vi "LVClass_WavefrontCorrector Assert Equal User Preferences.vi"(0 "WavefrontCorrector in":refnum<class "WavefrontCorrector.lvclass">, 5 "Wavefront Corrector State":T1[](array[typedef]), 7 "Sleep after command apply (ms)":i32, 11 "error in (no error)":errorcluster) -> (4 "WavefrontCorrector out":refnum<class "WavefrontCorrector.lvclass">, 15 "error out":errorcluster)   [LabVIEW 2020, in "WavefrontCorrector.lvclass"]
doc: "Assert requested preferences are equal to current preferences.\n\n--------------------------------------------------------------------------------\n\n<B>correctorIn </B> : WavefrontCorrector object.\n<B>correctorOut </B> : WavefrontCorrector object.\n<B>sleep_after_movement </B> : WavefrontCorrector preferences : Time to stabilization (ms).\n<B>min </B> : WavefrontCorrector preferences : lowest command value.\n<B>max </B> : WavefrontCorrector preferences : highest command value.\n<B>validity </B> : WavefrontCorrector preferences : status.\n<B>fixed_values </B> : WavefrontCorrector preferences : fixed positions.\n<B>ErrorIn </B> : Error\n<B>ErrorOut </B> : Error\n\n--------------------------------------------------------------------------------"
uses:
  WavefrontCorrector.lvclass
  Wavefront Corrector states - ONE.ctl
  WavefrontCorrector.lvclass/WavefrontCorrector.ctl
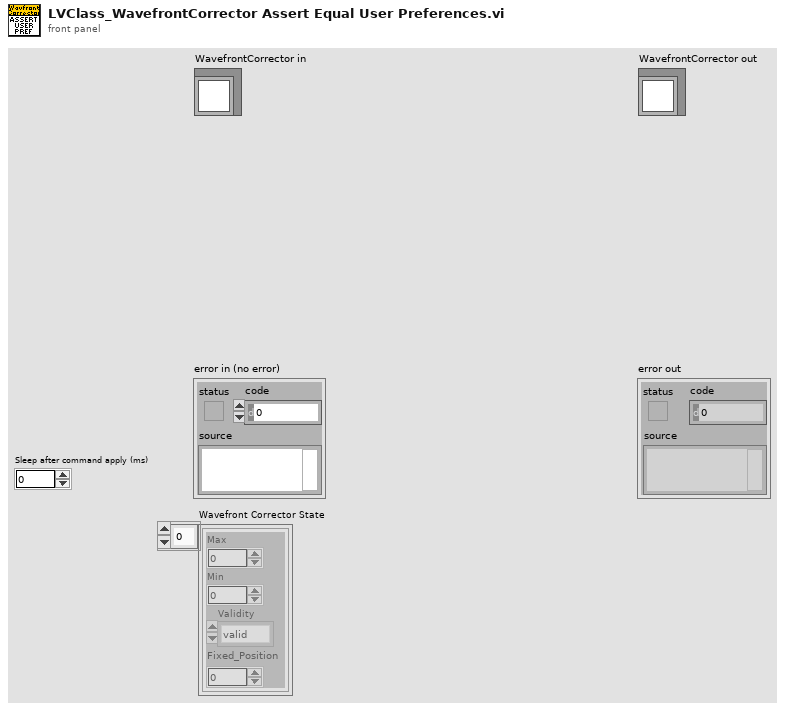
[diagram p1: front panel]
types:
  T1 = typedef "Wavefront Corrector states - ONE.ctl" = cluster{"Max":sgl, "Min":sgl, "Validity":enum16{"valid", "fixed", "invalid"}, "Fixed_Position":sgl}
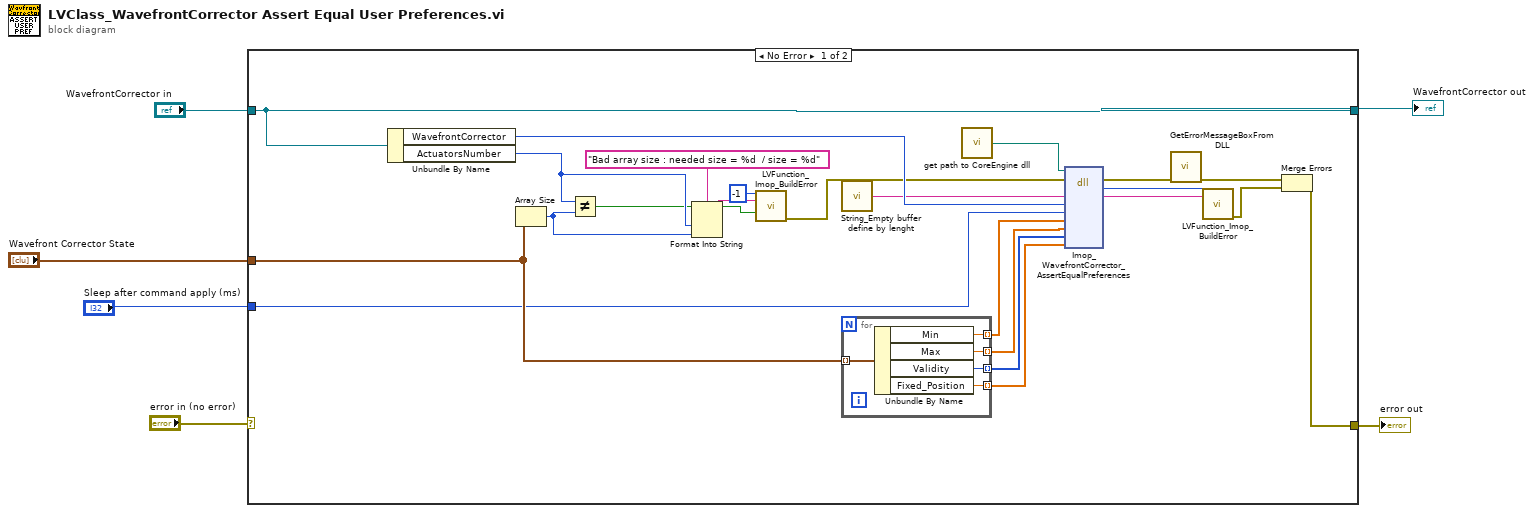
[diagram p0: block diagram]
diagram:
  n1 = case shown="No Error" "error in (no error)" {
    selector: "error in (no error)" -> [_ w36]
    tunnel: [w27 w36] -> w3
    tunnel: [w7 w35] -> w4
    tunnel: "WavefrontCorrector in" -> [w7 w35]
    tunnel: "Wavefront Corrector State" -> [w9 _]
    tunnel: "Sleep after command apply (ms)" -> [w8 _]
    frame No Error {
      n2 = Unbundle By Name(w7) -> ("WavefrontCorrector"=w26:i32, "ActuatorsNumber"=w19:i32)
      n3 = Array Size(array=w9) -> (size(s)=w20:i32)
      n4 = Not Equal?(x=w19, y=w20) -> (x != y?=w14:bool)
      n5 = Format Into String(format string="Bad array size : needed size = %d  / size = %d" ("String to Prepend to source (\"\")"), w19, w20) -> (resulting string=w21:string)  [unwired: 2 in, 1 out]
      n6 = call "LVFunction_Imop_BuildError.vi"("code"=-1, "String to Prepend to source (\"\")"=w21, "Activate error? (true)"=w14) -> ("error out"=w12:errorcluster)  [unwired: 12 in]
      n7 = call "String_Empty buffer define by lenght.vi"() -> ("Empty buffer"=w17:string)  [unwired: 1 in]
      n8 = for {
        tunnel: w9 -> [w34] mode=indexing
        tunnel: [w33] -> w11 mode=indexing
        tunnel: [w32] -> w10 mode=indexing
        tunnel: [w31] -> w16 mode=indexing
        tunnel: [w30] -> w15 mode=indexing
        n9 = Unbundle By Name(w34) -> ("Min"=w33:sgl, "Max"=w32:sgl, "Validity"=w31:enum16{"valid", "fixed", "invalid"}, "Fixed_Position"=w30:sgl)
      }
      n10 = call "get path to CoreEngine dll.vi"() -> ("path to c_interface_vc100.dll"=w18:path)  [unwired: 12 in, 3 out]
      n11 = dll-call lib="D:/soft/HASO_v3/SVN_trunk/ImOpCoreEngine4_LV2011/DLLs/c_interface_vc100.dll" fn="Imop_WavefrontCorrector_AssertEqualPreferences"(path in=w18, error in=w12, "message"=w17, "WavefrontCorrection"=w26, "sleep_after_movement"=w8, "min"=w11, "max"=w10, "validity"=w16, "fixed_value"=w15) -> (error out=w25:errorcluster, "return type"=w24:i32, "message"=w23:string)  [unwired: 7 in, 1 out]
      n12 = call "GetErrorMessageBoxFromDLL.vi"("error IN"=w25) -> ("error OUT"=w29:errorcluster)  [unwired: 10 in]
      n13 = call "LVFunction_Imop_BuildError.vi"("code"=w24, "String to Prepend to source (\"\")"=w23) -> ("error out"=w28:errorcluster)  [unwired: 13 in]
      n14 = Merge Errors(w29, w28) -> (w27:errorcluster)
    }
    frame Error {
    }
  }
  "error out" <- w3
  "WavefrontCorrector out" <- w4
